vi "PROGRAM_9.vi"() -> ()   [LabVIEW 2011]
panel:
  out "SUMA150":dbl
  out "Contador":dbl
  out "Velocidad promedio":dbl
  out "Velocidad":dbl(knob) scale=0.0..220.0
  # "GENERAR 10 PRUEBAS DE VELOCIDAD \nLUAGO SUMAR LAS VELOCIDADES\nMAYORES A 150 Y OBTENER SU PROMEDIO"
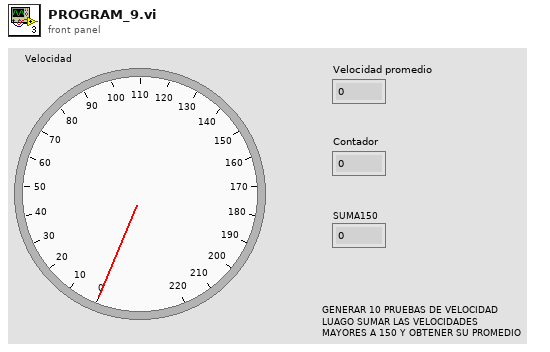
[diagram p1: front panel]
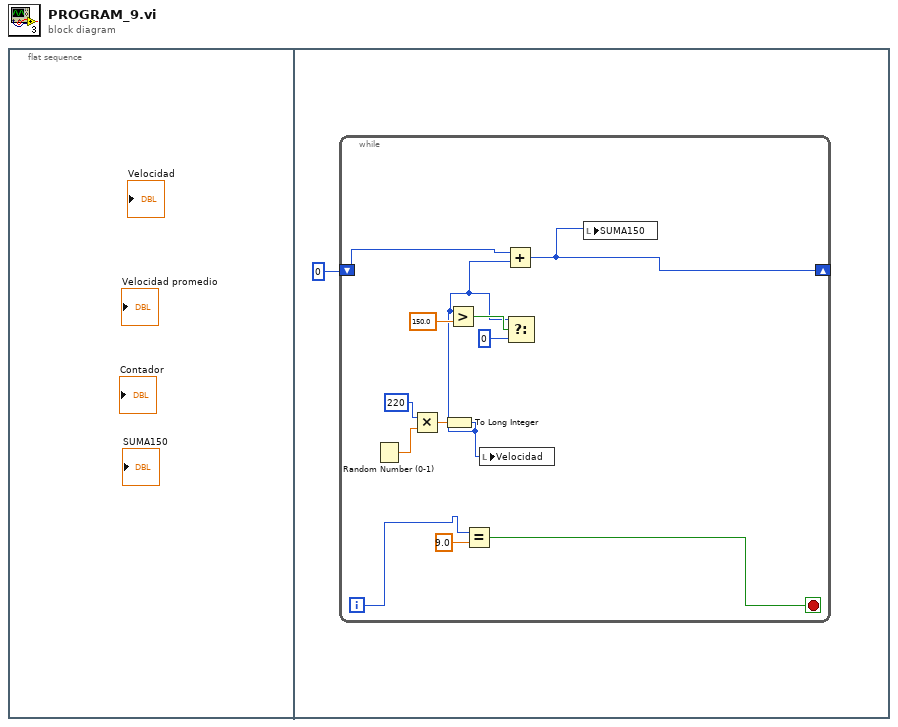
[diagram p0: block diagram]
diagram:
  n1 = flat-sequence {
    frame #0 {
    }
    frame #1 {
      n2 = while {
        shift-right: [w5] -> _
        shift-left: 0 -> [w13]
        i -> [w3]
        stop <- w2 stop-if-true
        n3 = Random Number (0-1)() -> (number: 0 to 1=w10:dbl)
        n4 = Multiply(x=220, y=w10) -> (x*y=w12:dbl)
        n5 = To Long Integer(number=w12) -> (32bit integer=w6:i32)
        n6 = Greater?(x=w6, y=150.0) -> (0:w8:bool)
        n7 = Equal?(x=w3, y=9.0) -> (x = y?=w2:bool)
        n8 = local write "Velocidad"(w6) -> ()
        n9 = Add(x=w13, y=w6) -> (x+y=w5:i32)
        n10 = Select(t=w6, s=w8, f=0) -> ()  [unwired: 1 out]
        n11 = local write "SUMA150"(w5) -> ()
      }
    }
  }
